vi "GetIMAQTimestamp.vi"(11 "Refnum in":T1) -> (3 "Time Stamp":timestamp)   [LabVIEW 2017, in "ImageAcquisitionLibrary.lvlib"]
uses:
  ImageAcquisitionLibrary.lvlib
  <vilib>/vision/Image Controls.llb/IMAQ Image.ctl
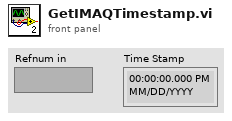
[diagram p1: front panel]
types:
  T1 = typedef "IMAQ Image.ctl" = refnum<image>
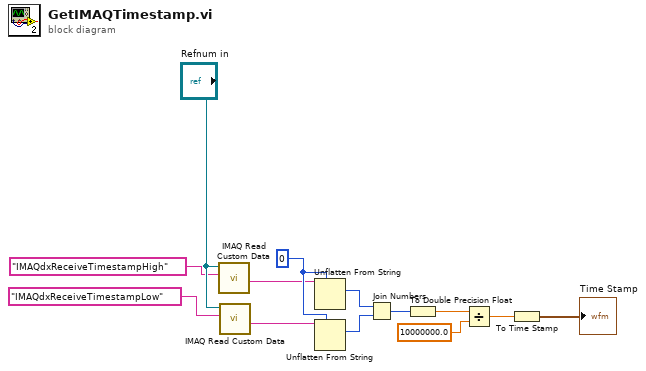
[diagram p0: block diagram]
diagram:
  w6 = 0
  n1 = call "IMAQ Read Custom Data"("Key"="IMAQdxReceiveTimestampHigh", "Image"="Refnum in") -> ("Custom Data Out"=w4:string)  [unwired: 7 in, 2 out]
  n2 = call "IMAQ Read Custom Data"("Key"="IMAQdxReceiveTimestampLow", "Image"="Refnum in") -> ("Custom Data Out"=w5:string)  [unwired: 7 in, 2 out]
  n3 = Unflatten From String(type=w6, binary string=w4) -> (value=w7:i32)  [unwired: 3 in, 2 out]
  n4 = Unflatten From String(type=w6, binary string=w5) -> (value=w8:i32)  [unwired: 3 in, 2 out]
  n5 = Join Numbers(hi=w7, lo=w8) -> ((hi.lo)=w12:u64)
  n6 = To Double Precision Float(number=w12) -> (double precision float=w9:dbl)
  n7 = Divide(x=w9, y=10000000.0) -> (x/y=w13:dbl)
  n8 = To Time Stamp(1:w13) -> (0:→"Time Stamp":timestamp)
